vi "Lex Reader.vi"(8 "Error In":errorcluster, 11 "Reader":refnum<class "Abstract.lvclass">) -> (0 "Error Out":errorcluster, 3 "Tokens":refnum<class "Abstract.lvclass">[](array[class]))   [LabVIEW 2018, in "Toolkit.lvlib"]
uses:
  Toolkit.lvlib
  Readers/Abstract/Abstract.lvclass
  Tokens/Abstract/Abstract.lvclass
  Lexer/Lexer.lvclass
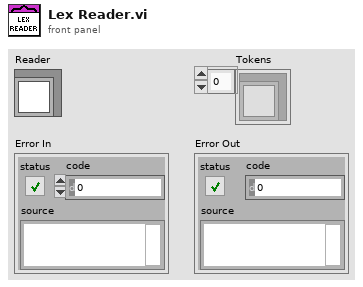
[diagram p1: front panel]
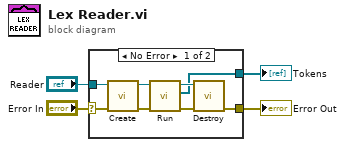
[diagram p0: block diagram]
diagram:
  n1 = case shown="No Error" "Error In" {
    selector: "Error In" -> [w6 w13]
    tunnel: "Reader" -> [w8 _]
    tunnel: [w7 _] -> w3
    tunnel: [w5 w13] -> w1
    frame No Error {
      n2 = call "Create.vi"("Error In"=w6, "Reader"=w8) -> ("Error Out"=w9:errorcluster, "Parser"=w12:refnum<class "Lexer.lvclass">)  [unwired: 8 in]
      n3 = call "Run.vi"("Error In"=w9, "Lexer In"=w12) -> ("Error Out"=w10:errorcluster, "Tokens"=w7:refnum<class "Abstract.lvclass">[], "Lexer Out"=w11:refnum<class "Lexer.lvclass">)  [unwired: 7 in]
      n4 = call "Destroy.vi"("Error In"=w10, "Parser"=w11) -> ("Error Out"=w5:errorcluster)  [unwired: 9 in]
    }
    frame Error {
    }
  }
  "Tokens" <- w3
  "Error Out" <- w1
